vi "Get Double Complex.vi"(7 "data type of variable":cdb, 8 "error in":errorcluster, 10 "variable name":string, 11 "GOLPI ref. in":T1={"pipe handle"={"lv_proc.dll file path"=path "", "process instance handle"=[]}, "fast read timeout [ms]"=500, "fast read settle time [ms]"=10, "fast read to multiple [ms]"=1, "max elements per input line"=100, "slow read timeout [ms]"=5000}) -> (0 "error out":errorcluster, 2 "value":cdb format="%.2f", 3 "GOLPI ref. out":T1={"pipe handle"={"lv_proc.dll file path"=path "", "process instance handle"=[]}, "fast read timeout [ms]"=500, "fast read settle time [ms]"=10, "fast read to multiple [ms]"=1, "max elements per input line"=100, "slow read timeout [ms]"=5000})   [LabVIEW 2013, in "GOLPI library.lvlib"]
uses:
  GOLPI library.lvlib
  Type Definitions/GOLPI reference Type Def.ctl
  LV Process.lvlibp/Pipe Handle.ctl
  Type Definitions/Custom Error Codes Enum Type Def.vi
  LV Process.lvlibp
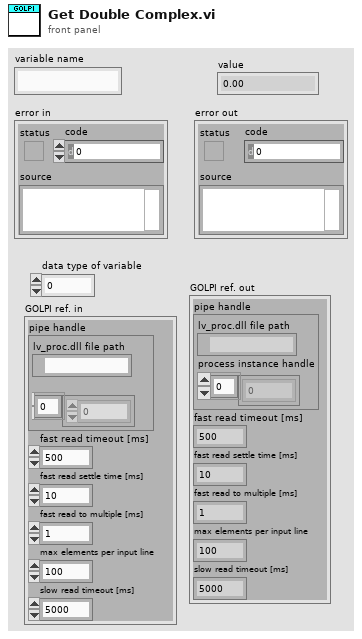
[diagram p1: front panel]
types:
  T1 = typedef "GOLPI library.lvlib/GOLPI reference Type Def.ctl" = cluster{"pipe handle":T2, "fast read timeout [ms]":u32, "fast read settle time [ms]":u32, "fast read to multiple [ms]":u32, "max elements per input line":u32, "slow read timeout [ms]":u32}
  T2 = typedef "LV Process.lvlibp/Pipe Handle.ctl" = cluster{"lv_proc.dll file path":path, "process instance handle":u32[]}
  T3 = typedef "GOLPI library.lvlib/Custom Error Codes Enum Type Def.vi" = enum16{"no error", "00 working directory PAR1 missing", "01 octave binary PAR1 missing", "02 octave report error PAR1", "03 empty output last cmd PAR1", "04 missing temporary file PAR1", "05 pwd PAR 1 not exist", "10 var PAR1 not string", "11 var PAR1 not num, scal, ~compl", "12 var PAR1 not num, scal, compl", "13 var PAR1 not num, vect, ~compl", "14 var PAR1 not num, vect, compl", "15 var PAR1 not num, mat, ~compl", "16 var PAR1 not num, mat, ~compl", "30 WARNING read timeout", "99 not finished"}
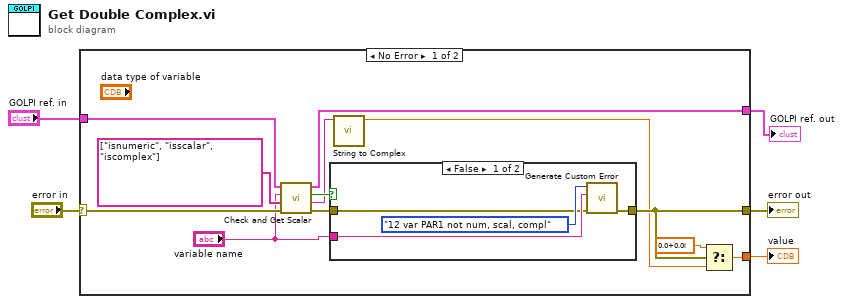
[diagram p0: block diagram]
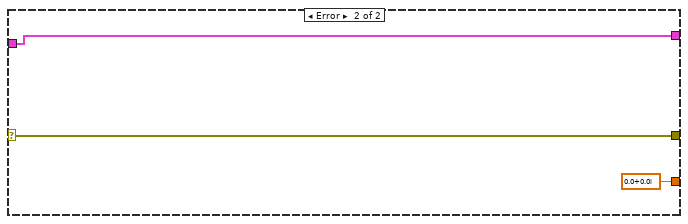
[diagram p3: hidden frame]
diagram:
  n1 = case shown="No Error" "error in" {
    selector: "error in" -> [w12 w25]
    tunnel: [w17 cdb 0.0+0.0i ("t")] -> w5
    tunnel: [w16 w25] -> w4
    tunnel: "GOLPI ref. in" -> [w7 w23]
    tunnel: [w6 w23] -> w1
    frame No Error {
      n2 = call "Check and Get Scalar.vi"("error in (no error)"=w12, "test commands"=string[] ["isnumeric", "isscalar", "iscomplex"], "variable name"="variable name", "GOLPI ref. in"=w7) -> ("error out"=w11:errorcluster, "variable"=w9:string, "all tests OK?"=w10:bool, "GOLPI ref. out"=w6:T1)  [unwired: 4 in]
      n3 = case shown="False" w10 {
        tunnel: [w18 w22] -> w16
        tunnel: w11 -> [w19 w22]
        tunnel: "variable name" -> [w20 _]
        frame False {
          n4 = call "Generate Custom Error.vi"("error in"=w19, "PAR1"=w20, "GOLPI error"=Custom_Error_Codes_Enum_Type_Def.vi."12 var PAR1 not num, scal, compl" ("Enum")) -> ("error out"=w18:errorcluster)  [unwired: 8 in]
        }
        frame True {
        }
      }
      n5 = call "String to Complex.vi"("string"=w9) -> ("complex number"=w14:cdb)  [unwired: 10 in]
      n6 = Select(t=cdb 0.0+0.0i, s=w16, f=w14) -> (s? t:f=w17:cdb)
    }
    frame Error {
    }
  }
  "value" <- w5
  "error out" <- w4
  "GOLPI ref. out" <- w1
